vi "wa32 Read Till Key.vi"(5 "include key in message (False)":bool, 7 "timeout [ms] (1000)":i32=1000, 8 "error in":errorcluster, 9 "max message length (1024)":i32=1024, 10 "key string":string, 11 "handle":i32) -> (0 "error out":errorcluster, 2 "read message":string, 3 "handle out":i32)   [LabVIEW 2020, in "GOLPI library.lvlib"]
doc: "This VI reads open handle till key string is found in the read data. It does not remove data from the pipe until the key is detected. Then it reads the message with the key and returns it either with or without the key. \nIf timeout is reached or maximum message size is reached the function will stop and return error.\nNote the function has internal latency around 50 ms."
uses:
  GOLPI library.lvlib
  <vilib>/Utility/error.llb/Error Cluster From Error Code.vi
  <vilib>/ErrorRing/Error Ring.xnode
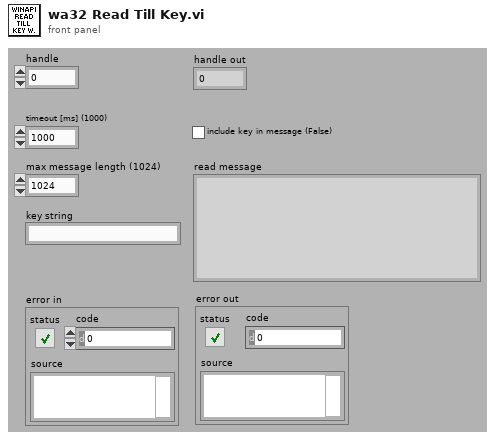
[diagram p1: front panel]
types:
  T1 = enum16{"Native", "Native Command Line", "UNIX", "Macintosh", "DOS"}
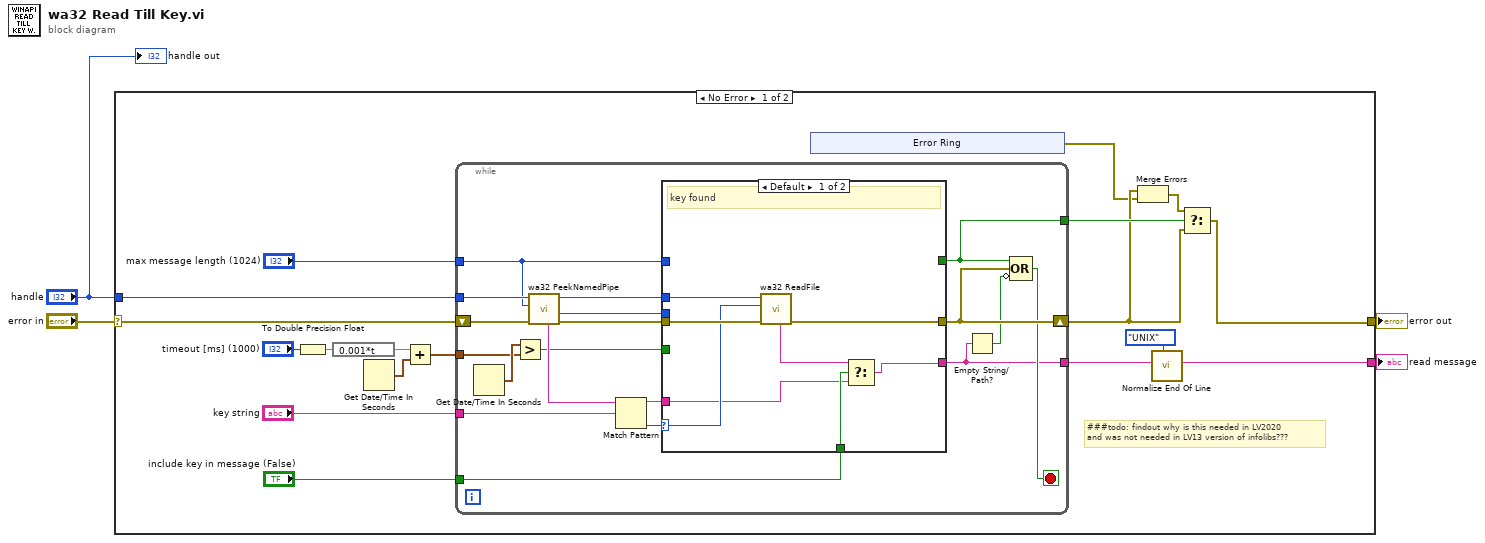
[diagram p0: block diagram]
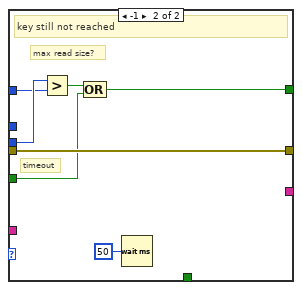
[diagram p2: hidden frame]
diagram:
  n1 = case shown="No Error" "error in" {
    selector: "error in" -> [w8 w62]
    tunnel: "handle" -> [w22 _]
    tunnel: [w6 _] -> w3
    tunnel: [w12 w62] -> w2
    frame No Error {
      # "###todo: findout why is this needed in LV2020\nand was not needed in LV13 version of infolibs???"
      n2 = To Double Precision Float(number="timeout [ms] (1000)") -> (double precision float=w18:dbl)
      n3 = expression code="0.001*t"(w18) -> (w17:dbl)
      n4 = Get Date/Time In Seconds() -> (seconds since 1Jan1904=w16:timestamp)
      n5 = Add(x=w17, y=w16) -> (x+y=w15:timestamp)
      n6 = while {
        tunnel: w22 -> [w45]
        tunnel: "key string" -> [w44]
        tunnel: "max message length (1024)" -> [w38]
        shift-right: [w34] -> w10
        shift-left: w8 -> [w46]
        tunnel: w15 -> [w36]
        tunnel: [w32] -> w14
        tunnel: [w30] -> w13
        tunnel: "include key in message (False)" -> [w29]
        stop <- w33 stop-if-true
        n7 = Get Date/Time In Seconds() -> (seconds since 1Jan1904=w37:timestamp)
        n8 = Greater?(x=w37, y=w36) -> (0:w35:bool)
        n9 = call "wa32 PeekNamedPipe.vi"("error in"=w46, "bytes to read (0)"=w38, "handle"=w45) -> ("error out"=w41:errorcluster, "read bytes"=w39:u32, "handle out"=w40:i32, "string data"=w43:string)  [unwired: 3 in, 2 out]
        n10 = Match Pattern(string=w43, regular expression=w44) -> (before substring=w28:string, offset past match=w42:i32)  [unwired: 1 in, 2 out]
        n11 = case shown="Default" w42 {
          selector: w42 -> [w48 _]
          tunnel: w41 -> [w54 w59]
          tunnel: w40 -> [w53 _]
          tunnel: w39 -> [_ w61]
          tunnel: w38 -> [_ w60]
          tunnel: [w52 w59] -> w34
          tunnel: w35 -> [_ w57]
          tunnel: [_ w56] -> w30
          tunnel: [w49 _] -> w32
          tunnel: w29 -> [w51 _]
          tunnel: w28 -> [w47 _]
          frame Default {
            # "key found"
            n12 = call "wa32 ReadFile.vi"("error in"=w54, "bytes to read (0)"=w48, "handle"=w53) -> ("error out"=w52:errorcluster, "read string"=w50:string)  [unwired: 4 in, 3 out]
            n13 = Select(t=w50, s=w51, f=w47) -> (s? t:f=w49:string)
          }
          frame -1 {
            # "timeout"
            # "max read size?"
            # "key still not reached"
            n14 = Greater?(x=w61, y=w60) -> (0:w58:bool)
            n15 = Compound Arithmetic op=OR(w58, w57) -> (w56:bool)
            n16 = Wait (ms)(milliseconds to wait=u32 50) -> ()  [unwired: 1 out]
          }
        }
        n17 = Empty String/Path?(string/path=w32) -> (empty?=w31:bool)
        n18 = Compound Arithmetic op=OR(w30, w34, invert w31) -> (w33:bool)
      }
      n19 = xnode "Error Ring"() -> ("error out"=w9:errorcluster)
      n20 = Merge Errors(w10, w9) -> (w11:errorcluster)
      n21 = call <vilib>:"Normalize End Of Line.vi"("end of line (Native)"=T1."UNIX", "string in"=w14) -> ("string out"=w6:string)  [unwired: 6 in]
      n22 = Select(t=w11, s=w13, f=w10) -> (s? t:f=w12:errorcluster)
    }
    frame Error {
    }
  }
  "read message" <- w3
  "error out" <- w2
  "handle out" <- "handle"
